vi "In_S7F19.vi"(8 "error in (no error)":errorcluster, 11 "S7 Message Class in":refnum<class "S7 Message Class.lvclass">) -> (0 "error out":errorcluster, 2 "OK?":bool, 3 "S7 Message Class out":refnum<class "S7 Message Class.lvclass">)   [LabVIEW 2020, in "SECS Communication.lvlib" / "S7 Message Class.lvclass"]
uses:
  S7 Message Class.lvclass
  D:/Dropbox/SECS/SECS_GEM v1.0.5/Com/SECS Communication/SECS-II Class/SECS-II Class.lvclass
  SECS-II Class/SECS-II Class.lvclass/SECS-II Class.ctl
  SECS-II Class/SECS-II Class.lvclass
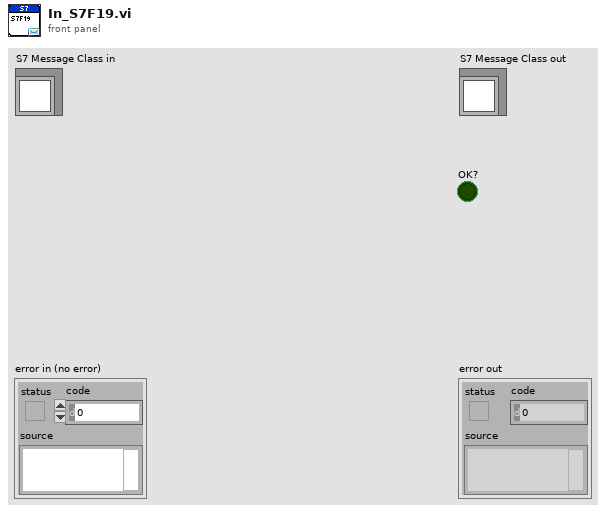
[diagram p1: front panel]
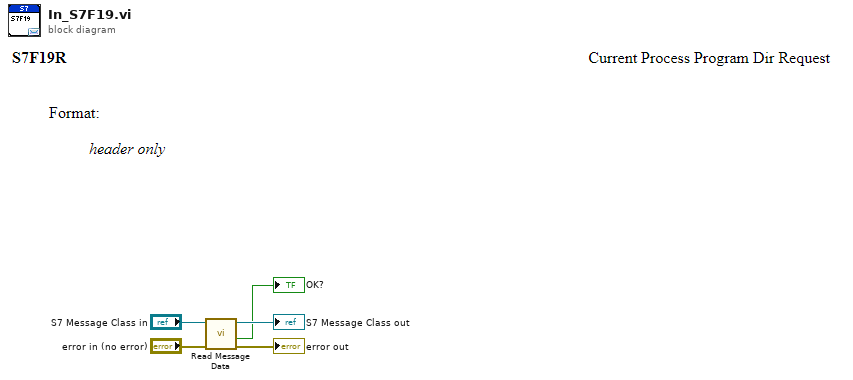
[diagram p0: block diagram]
diagram:
  n1 = call "Read Message Data.vi"("error in (no error)"="error in (no error)", "SECS-II Class in"="S7 Message Class in") -> ("error out"=→"error out":errorcluster, "Empty?"=→"OK?":bool, "SECS-II Class out"=→"S7 Message Class out":refnum<class "S7 Message Class.lvclass">)  [unwired: 6 in, 1 out]
